vi "Deadzone.vi"(2 "Joystick Value Input":dbl, 3 "Deadzone Size":dbl) -> (0 "Corrected Joystick Value":dbl)   [LabVIEW 2020]
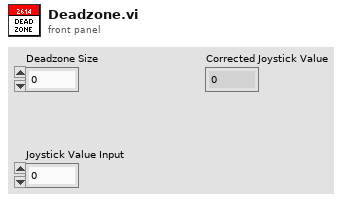
[diagram p1: front panel]
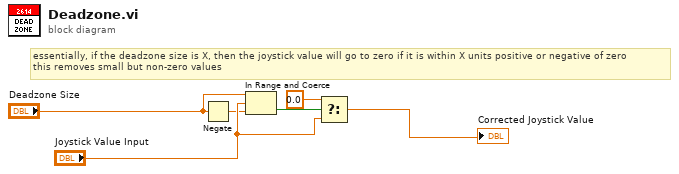
[diagram p0: block diagram]
diagram:
  # "essentially, if the deadzone size is X, then the joystick value will go to zero if it is within X units positive or negative of zero\nthis removes small but non-zero values"
  n1 = Negate(x="Deadzone Size") -> (-x=w2:dbl)
  n2 = In Range and Coerce(upper limit="Deadzone Size", x="Joystick Value Input", lower limit=w2) -> (In Range?=w3:bool)  [unwired: 1 out]
  n3 = Select(t=0.0, s=w3, f="Joystick Value Input") -> (s? t:f=→"Corrected Joystick Value":dbl)
